vi "Insert new data in histograms.vi"(8 "Error in":errorcluster, 9 "Seconds between updates":i32, 10 "Coincidences":T2[](array[typedef]), 11 "Cluster":T1) -> (0 "error out":errorcluster, 3 "Cluster":T1)   [LabVIEW 2016]
uses:
  Typedefs/Coincidence.ctl
  Typedefs/Coincidence histogram cluster refnum.ctl
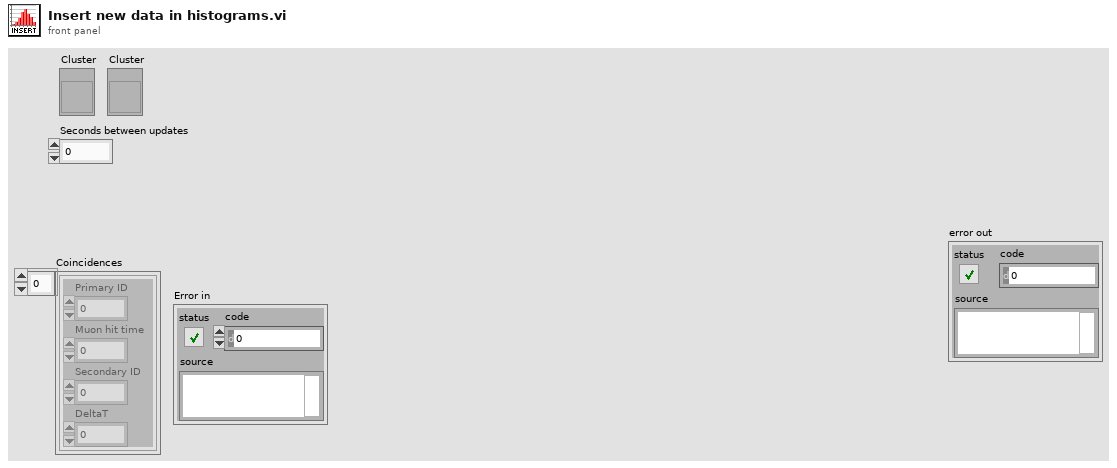
[diagram p1: front panel]
types:
  T1 = typedef "Coincidence histogram cluster refnum.ctl" = refnum<vi>
  T2 = typedef "Coincidence.ctl" = cluster{"Primary ID":i8, "Muon hit time":u64, "Secondary ID":i8, "DeltaT":i32}
  T3 = cluster{"Primary ID":i8, "Secondary ID":i8, "Data":i32[]}[]
  T4 = typedef "Semaphore RefNum" = refnum<k1>
  T5 = typedef "Coincidence single histogram.ctl" = cluster{"Histogram Graph":cluster{"X Values":dbl[], "Histogram: h(x)":i32[]}[], "IDs":i8[], "Datapoints:":i32, "S:":dbl, "Data array":cluster{"Data":i32[], "Max index":i32, "Current index":i32, "Numofpoints":i32}}
  T6 = cluster{"X Values":dbl[], "Histogram: h(x)":i32[]}[]
  T7 = cluster{"Data":i32[], "Max index":i32, "Current index":i32, "Numofpoints":i32}
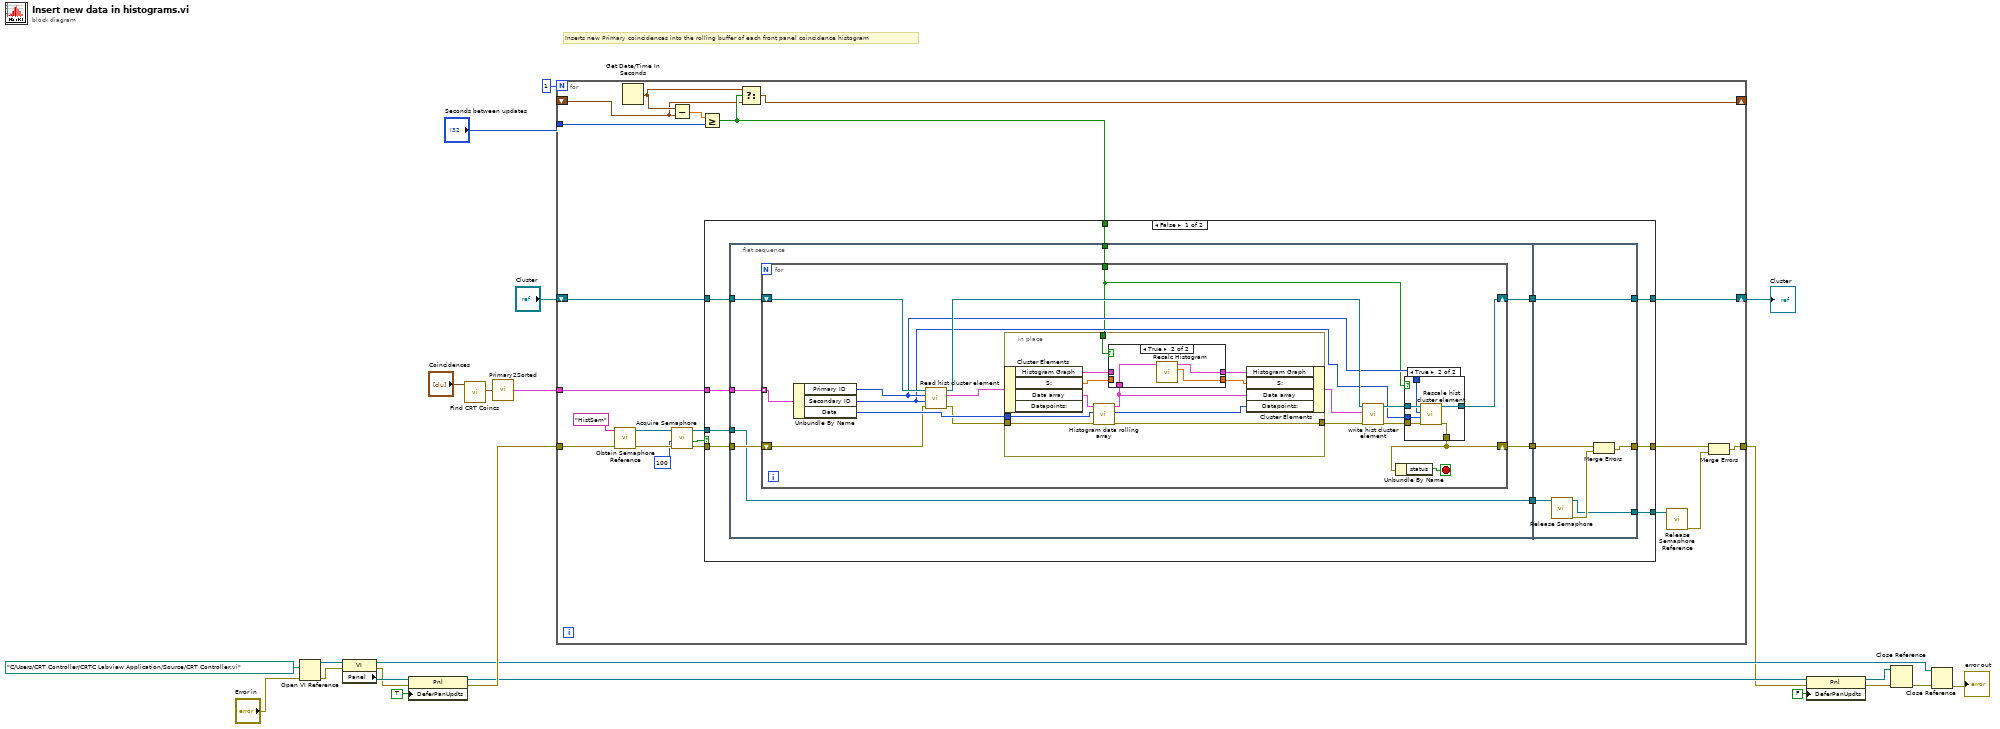
[diagram p0: block diagram]
diagram:
  # "Inserts new Primary coincidences into the rolling buffer of each front panel coincidence histogram"
  n1 = Open VI Reference(vi path=path "C:/Users/CRT Controller/CRTC Labview Application/Source/CRT Controller.vi", error in (no error)="Error in") -> (vi reference=w20:refnum<vi>, error out=w19:errorcluster)  [unwired: 4 in]
  n2 = property class="VI"(reference=w20, error in=w19) -> (reference out=w7:refnum<vi>, error out=w15:errorcluster, "Panel"=w17:refnum<vi>)
  n3 = property class="Pnl"(reference=w17, error in=w15, "DeferPanUpdts"=TRUE ("Defer Panel Updates")) -> (reference out=w12:refnum<vi>, error out=w13:errorcluster)
  n4 = call "Find CRT Coincs.vi"("Coincidences"="Coincidences") -> ("Single hits"=w1:T2[])  [unwired: 8 in, 2 out]
  n5 = call "Primary2Sorted.vi"("Primary channel coincidences"=w1) -> ("Sorted data"=w23:T3)
  n6 = for {
    N: 1 -> [_]
    tunnel: w23 -> [w44]
    tunnel: w13 -> [w34]
    tunnel: [w24] -> w6
    shift-right: [w38] -> _
    shift-left: _ -> [w39]
    tunnel: "Seconds between updates" -> [w42]
    shift-right: [w36] -> w3
    shift-left: "Cluster" -> [w37]
    n7 = call <vilib>:"Obtain Semaphore Reference.vi"("error in (no error)"=w34, "name (unnamed)"="HistSem") -> ("error out"=w32:errorcluster, "semaphore"=w33:T4)  [unwired: 3 in, 1 out]
    n8 = Get Date/Time In Seconds() -> (seconds since 1Jan1904=w40:timestamp)
    n9 = Subtract(x=w40, y=w39) -> (x-y=w43:dbl)
    n10 = call <vilib>:"Acquire Semaphore.vi"("error in (no error)"=w32, "ms timeout (-1)"=100, "semaphore"=w33) -> ("error out"=w31:errorcluster, "timed out"=w29:bool, "semaphore out"=w28:T4)  [unwired: 2 in]
    n11 = Greater Or Equal?(x=w43, y=w42) -> (x >= y?=w41:bool)
    n12 = case shown="False" w29 {
      tunnel: w44 -> [w55 _]
      tunnel: [w48 w111] -> w26
      tunnel: w41 -> [w54 _]
      tunnel: w37 -> [w53 w110]
      tunnel: [w52 w110] -> w36
      tunnel: w31 -> [w51 w111]
      tunnel: w28 -> [w46 w112]
      tunnel: [w47 w112] -> w27
      frame False {
        n13 = flat-sequence {
          tunnel: w55 -> [w62]
          tunnel: w54 -> [w61]
          tunnel: w53 -> [w60]
          tunnel: w51 -> [w58]
          tunnel: [w59] -> w50
          tunnel: [w57] -> w49
          tunnel: w46 -> [w56]
          tunnel: [w56] -> w45
          tunnel: [w109] -> w52
          tunnel: w50 -> [w109]
          tunnel: w49 -> [w107]
          tunnel: [w106] -> w48
          tunnel: [w105] -> w47
          tunnel: w45 -> [w104]
          frame #0 {
            n14 = for {
              tunnel: w62 -> [w79] mode=indexing
              shift-right: [w66] -> w57
              shift-left: w58 -> [w77]
              tunnel: w61 -> [w64]
              shift-right: [w65] -> w59
              shift-left: w60 -> [w75]
              stop <- w76 stop-if-true
              n15 = Unbundle By Name(w79) -> ("Primary ID"=w69:i8, "Secondary ID"=w68:i8, "Data"=w78:i32[])
              n16 = call "Read hist cluster element.vi"("error in (no error)"=w77, "Secondary"=w68, "Primary"=w69, "histogram in"=w75) -> ("error out"=w73:errorcluster, "histogram"=w74:T5, "histogram out"=w71:T1)  [unwired: 5 in]
              n17 = in-place {
                in-place-border: w73 -> [w98]
                in-place-border: [w97] -> w72
                in-place-border: w64 -> [w93]
                in-place-border: w78 -> [w92]
                n18 = in-place-cluster #1(w74) -> ("Histogram Graph"=w89:T6, "S:"=w88:dbl, "Data array"=w96:T7)  [unwired: 1 out]
                n19 = call "Histogram data rolling array.vi"("error in (no error)"=w98, "new data"=w92, "Rolling array in"=w96) -> ("error out"=w97:errorcluster, "Numofpoints"=w95:i32, "Rolling array out"=w94:T7)  [unwired: 6 in]
                n20 = case shown="True" w93 {
                  tunnel: w94 -> [_ w103]
                  tunnel: [w100 w102] -> w91
                  tunnel: w89 -> [w100 _]
                  tunnel: [w99 w101] -> w90
                  tunnel: w88 -> [w99 _]
                  frame False {
                  }
                  frame True {
                    n21 = call "Recalc Histogram.vi"("Rolling array in"=w103) -> ("standard deviation"=w101:dbl, "Hist and fit"=w102:T6)  [unwired: 9 in]
                  }
                }
                n22 = in-place-cluster #1("Histogram Graph"=w91, "S:"=w90, "Data array"=w94, "Datapoints:"=w95) -> (w63:T5)
              }
              n23 = call "write hist cluster element.vi"("error in (no error)"=w72, "histogram"=w63, "Hist cluster"=w71) -> ("error out"=w67:errorcluster, "Hist cluster"=w70:T1)  [unwired: 7 in]
              n24 = case shown="True" w64 {
                tunnel: w70 -> [w80 w87]
                tunnel: w69 -> [_ w86]
                tunnel: w68 -> [_ w85]
                tunnel: w67 -> [w81 w84]
                tunnel: [w81 w83] -> w66
                tunnel: [w80 w82] -> w65
                frame False {
                }
                frame True {
                  n25 = call "Rescale hist cluster element.vi"("error in (no error)"=w84, "Secondary"=w85, "Primary"=w86, "Hist cluster"=w87) -> ("error out"=w83:errorcluster, "Hist cluster"=w82:T1)  [unwired: 6 in]
                }
              }
              n26 = Unbundle By Name(w66) -> ("status"=w76:bool)
            }
          }
          frame #1 {
            n27 = call <vilib>:"Release Semaphore.vi"("semaphore"=w104) -> ("error out"=w108:errorcluster, "semaphore out"=w105:T4)  [unwired: 5 in]
            n28 = Merge Errors(w107, w108) -> (w106:errorcluster)
          }
        }
      }
      frame True {
      }
    }
    n29 = Select(t=w40, s=w41, f=w39) -> (s? t:f=w38:timestamp)
    n30 = call <vilib>:"Release Semaphore Reference.vi"("semaphore"=w27) -> ("error out"=w25:errorcluster)  [unwired: 9 in, 1 out]
    n31 = Merge Errors(w26, w25) -> (w24:errorcluster)
  }
  "Cluster" <- w3
  n32 = property class="Pnl"(reference=w12, error in=w6, "DeferPanUpdts"=FALSE ("Defer Panel Updates")) -> (reference out=w9:refnum<vi>, error out=w10:errorcluster)
  n33 = Close Reference(reference=w9, error in (no error)=w10) -> (error out=w8:errorcluster)
  n34 = Close Reference(reference=w7, error in (no error)=w8) -> (error out=→"error out":errorcluster)
